vi "test_Create Global MetaData Channel_array enumerated list.vi"(8 "error in (no error)":errorcluster, 11 "TestCase in":refnum<class "Instrument Addon Scripting API Channels Unit Tests.lvclass">) -> (0 "error out":errorcluster, 3 "TestCase out":refnum<class "Instrument Addon Scripting API Channels Unit Tests.lvclass">)   [LabVIEW 2018, in "Instrument Addon Scripting API Channels Unit Tests.lvclass"]
uses:
  Instrument Addon Scripting API Channels Unit Tests.lvclass
  Addon/Addon Shared/Types/FG Control.ctl
  APIs/Scripting API/TypeDefs/Array Enumerated List Settings.ctl
  APIs/Scripting API/TypeDefs/Array Element.ctl
  Instrument Addon Scripting API Channels Unit Tests.lvclass/Instrument Addon Scripting API Channels Unit Tests.ctl
  Addon/Addon Shared/SubVIs/Constants.vi
  APIs/Scripting API/Channels/Create Global MetaData Channel - Array - Enumerated List.vi
  <vilib>/NI Veristand/Custom Device Tools/Custom Device Utility Library/NI VeriStand - Search for Item by GUID.vi
  <vilib>/NI Veristand/Custom Device Tools/Custom Device Utility Library/NI VeriStand - Search for Item by Name.vi
  <vilib>/NI Veristand/Custom Device API/NI VeriStand - Get Item Property.vi
  <vilib>/NI Veristand/Custom Device API/Get Item Property (U32).vi
  <vilib>/NI Veristand/Custom Device API/Get Item Property (String Array).vi
  <vilib>/NI Veristand/Custom Device API/Get Item Property (String).vi
  <vilib>/NI Veristand/Custom Device API/NI VeriStand - Set Item Property.vi
  <vilib>/NI Veristand/Custom Device API/Set Item Property (U32).vi
  <vilib>/NI Veristand/Custom Device API/Set Item Property (String Array).vi
  <vilib>/NI Veristand/Custom Device API/NI VeriStand - Get Item Children.vi
  Addon/Addon Shared/SubVIs/Set Channel Value Table.vi
  <vilib>/NI Veristand/Custom Device API/Set Item Property (String).vi
  <vilib>/addons/_JKI Toolkits/VI Tester/TestCase.llb/TestCase.lvclass
  Instrument Addon Scripting API Test Assets/Instrument Addon Scripting API Test Assets.lvclass
  <vilib>/NI Veristand/Custom Device Tools/Custom Device Utility Library/Custom Device Utility Library.lvlib
  Addon/Addon Shared/Instrument Addon Shared.lvlib
  APIs/Scripting API/Instrument Addon Scripting API.lvlib
  C:/Program Files (x86)/National Instruments/LabVIEW 2018/vi.lib/addons/_JKI Toolkits/VI Tester/TestCase.llb/TestCase.lvclass
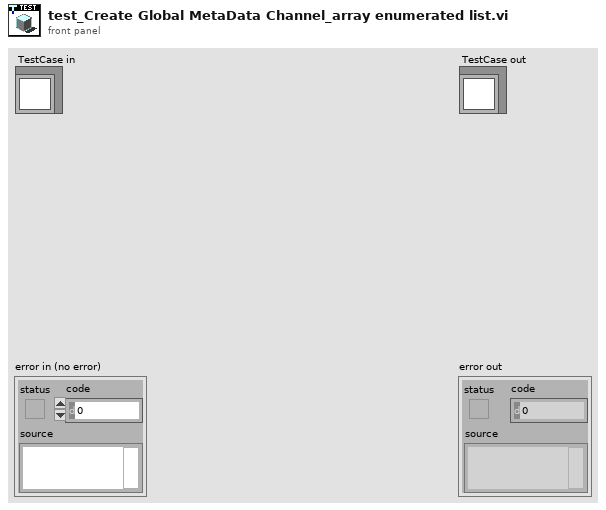
[diagram p1: front panel]
types:
  T1 = typedef "Instrument Addon Shared.lvlib/FG Control.ctl" = enum16{"Get", "Set"}
  T2 = typedef "Instrument Addon Scripting API.lvlib/Array Enumerated List Settings.ctl" = cluster{"Elements":T3[], "Enumerated List":string[], "Delimiter":string}
  T3 = typedef "Instrument Addon Scripting API.lvlib/Array Element.ctl" = cluster{"Name":string, "Default Value":dbl, "Units":string}
  T4 = typedef "Custom Device API.lvlib/Custom Device Item Ref.ctl" = u64
  T5 = typedef "Instrument Addon Shared.lvlib/MetaData Parameters.ctl" = cluster{"Data Type":T6, "Channel Type":T7, "List":string[], "Format String":string, "Type":T8, "Delimiter":string, "Endian":T9}
  T6 = typedef "Instrument Addon Shared.lvlib/Protocol Data Type.ctl" = enum16{"Single Channel", "Array"}
  T7 = typedef "Instrument Addon Shared.lvlib/Metadata Channel Type.ctl" = enum16{"Enumerated List", "Format", "Type Cast"}
  T8 = typedef "Instrument Addon Shared.lvlib/Type Cast Type.ctl" = enum16{"DBL", "SGL", "U64", "U32", "U16", "U8", "I64", "I32", "I16", "I8"}
  T9 = typedef "Instrument Addon Shared.lvlib/Endian.ctl" = enum16{"Native", "Little", "Big"}
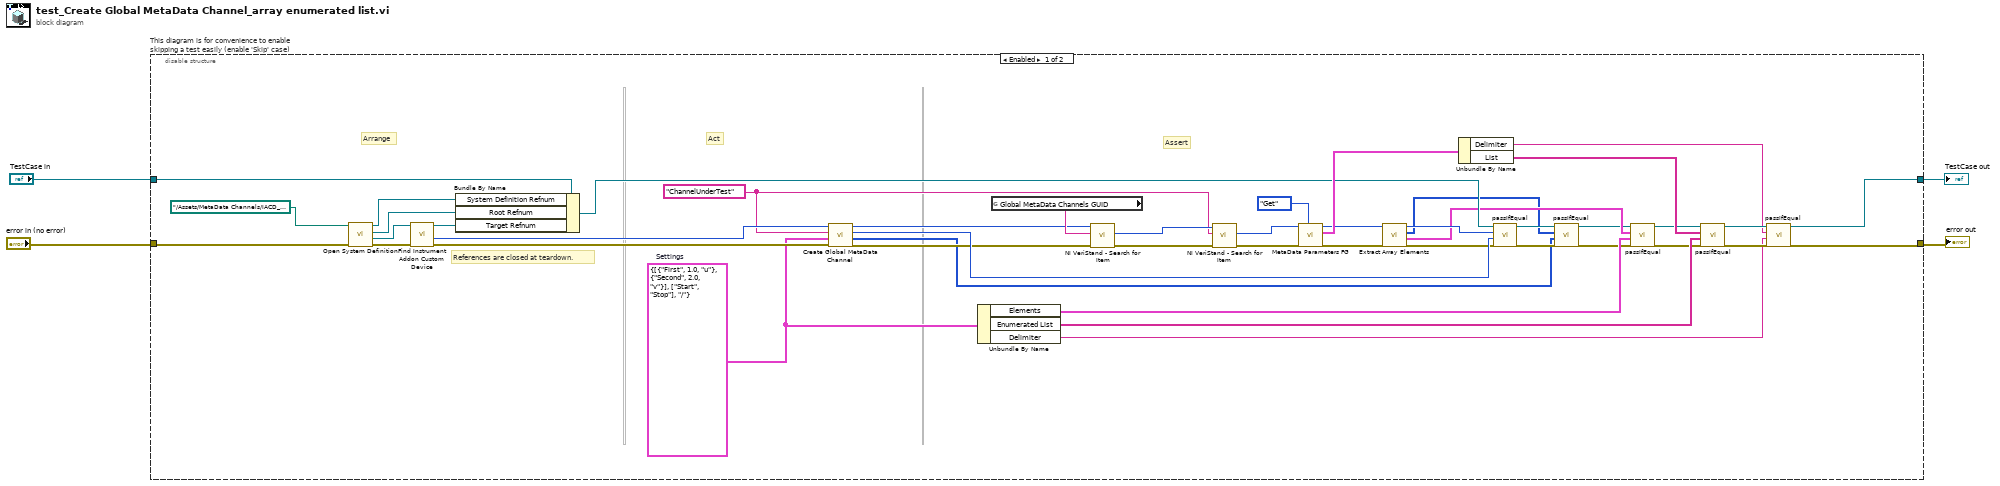
[diagram p0: block diagram]
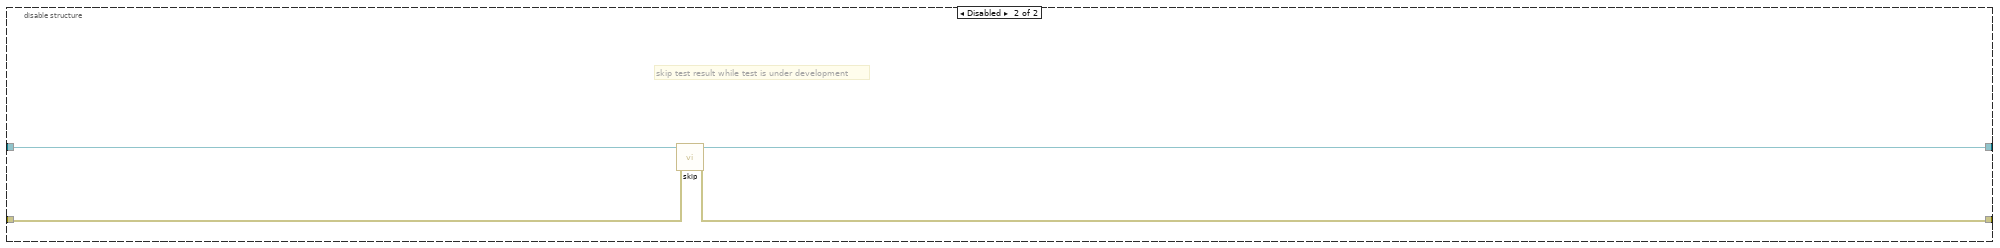
[diagram p2: hidden frame]
diagram:
  n1 = disable-structure "This diagram is for convenience to enable skipping a test easily (enable 'Skip' case)" shown="Enabled" {
    disable-tunnel: "TestCase in" -> [w31 w53]
    disable-tunnel: [w21 w51] -> w1
    disable-tunnel: [w20 w52] -> w3
    disable-tunnel: "error in (no error)" -> [w49 w50]
    frame Enabled {
      w24 = T2 {"Elements"=[{"Name"="First", "Default Value"=1.0, "Units"="u"}, {"Name"="Second", "Default Value"=2.0, "Units"="v"}], "Enumerated List"=["Start", "Stop"], "Delimiter"="/"}  # Settings
      w29 = "ChannelUnderTest" ("Name")
      # "References are closed at teardown."
      # "Assert"
      # "Act"
      # "Arrange"
      n2 = call "Open System Definition.vi"("error in (no error)"=w49, "System Definition File"=path "../Assets/MetaData Channels/IACD_channels.nivssdf") -> ("error out"=w47:errorcluster, "Target Refnum"=w48:refnum<k24>, "Root Refnum"=w34:refnum<k24>, "System Definition Refnum"=w33:refnum<k24>)  [unwired: 6 in]
      n3 = call "Find Instrument Addon Custom Device.vi"("error in"=w47, "target in"=w48) -> ("error out"=w28:errorcluster, "NodeID"=w30:u64, "target out"=w35:refnum<k24>)  [unwired: 7 in]
      n4 = Bundle By Name(cluster=w31, "System Definition Refnum"=w33, "Root Refnum"=w34, "Target Refnum"=w35) -> (w32:refnum<class "Instrument Addon Scripting API Channels Unit Tests.lvclass">)
      n5 = call-poly "Create Global MetaData Channel.vi"("Error In"=w28, "Settings"=w24, "Name"=w29, "Instrument Addon Refnum In"=w30) -> ("Error Out"=w25:errorcluster, "Channel Refnums"=w6:T4[], "Array Refnum"=w26:T4, "Instrument Addon Refnum Out"=w27:T4)  [unwired: 4 in]
      n6 = Unbundle By Name(w24) -> ("Elements"=w17:T3[], "Enumerated List"=w36:string[], "Delimiter"=w23:string)
      n7 = global read "Constants.vi" "Global MetaData Channels GUID"() -> (w46:string)
      n8 = call-poly <vilib>:"NI VeriStand - Search for Item.vi"("error in"=w25, "Item GUID"=w46, "Section Ref in"=w27) -> ("error out"=w44:errorcluster, "Item Ref"=w45:T4)  [unwired: 5 in, 2 out]
      n9 = call-poly <vilib>:"NI VeriStand - Search for Item.vi"("error in"=w44, "Item Name"=w29, "Section Ref in"=w45) -> ("error out"=w43:errorcluster, "Item Ref"=w42:T4)  [unwired: 5 in, 2 out]
      n10 = call "MetaData Parameters FG.vi"("Action"=FG_Control."Get", "error in (no error)"=w43, "Item Ref in"=w42) -> ("error out"=w16:errorcluster, "MetaData Parameters"=w40:T5, "Item Ref out"=w15:T4)  [unwired: 6 in]
      n11 = call "Extract Array Elements.vi"("error in (no error)"=w16, "array reference in"=w15) -> ("error out"=w14:errorcluster, "elements"=w12:T3[], "channel refnums"=w7:T4[], "array reference out"=w13:T4)  [unwired: 6 in]
      n12 = Unbundle By Name(w40) -> ("Delimiter"=w22:string, "List"=w37:string[])
      n13 = call-dynamic "passIfEqual.vi"("error in (no error)"=w14, "y"=w26, "x"=w13, "TestCase in"=w32) -> ("error out"=w11:errorcluster, "TestCase out"=w9:refnum<class "Instrument Addon Scripting API Channels Unit Tests.lvclass">)  [unwired: 6 in]
      n14 = call-dynamic "passIfEqual.vi"("error in (no error)"=w11, "y"=w6, "x"=w7, "TestCase in"=w9) -> ("error out"=w10:errorcluster, "TestCase out"=w8:refnum<class "Instrument Addon Scripting API Channels Unit Tests.lvclass">)  [unwired: 6 in]
      n15 = call-dynamic "passIfEqual.vi"("error in (no error)"=w10, "y"=w17, "x"=w12, "TestCase in"=w8) -> ("error out"=w18:errorcluster, "TestCase out"=w19:refnum<class "Instrument Addon Scripting API Channels Unit Tests.lvclass">)  [unwired: 6 in]
      n16 = call-dynamic "passIfEqual.vi"("error in (no error)"=w18, "y"=w36, "x"=w37, "TestCase in"=w19) -> ("error out"=w39:errorcluster, "TestCase out"=w38:refnum<class "Instrument Addon Scripting API Channels Unit Tests.lvclass">)  [unwired: 6 in]
      n17 = call-dynamic "passIfEqual.vi"("error in (no error)"=w39, "y"=w23, "x"=w22, "TestCase in"=w38) -> ("error out"=w20:errorcluster, "TestCase out"=w21:refnum<class "Instrument Addon Scripting API Channels Unit Tests.lvclass">)  [unwired: 6 in]
    }
    frame Disabled {
      # "skip test result while test is under development"
      n18 = call <vilib>:"skip.vi"("error in (no error)"=w50, "TestCase in"=w53) -> ("error out"=w52:errorcluster, "TestCase out"=w51:refnum<class "Instrument Addon Scripting API Channels Unit Tests.lvclass">)  [unwired: 8 in]
    }
  }
  "error out" <- w3
  "TestCase out" <- w1
